vi "SVA 4MV6 T027 CCE.vi"(7 "NORMALIZACIÓN":bool, 8 "INVERTIDO?":bool, 9 "UMBRAL":u8(knob) scale=0.0..255.0, 10 "CAPA DE COLOR":T1(ring), 11 "RUTA DE IMAGEN":path) -> (2 "MOMENTOS INVARIANTES DE HU":dbl[](array[numeric]), 3 "IMAGEN BINARIZADA":picture)   [LabVIEW 2020]
doc: "Ceballos Conde Emanuel 4MV6 Sistemas de visión artificial 2022/1\nEste vi permite obtener una imagen binarizada y LOS SIETE MOMENTOS INVARIANTES DE HU de una imagen, tomando como referencia una de las capas seleccionadas."
panel:
  # "Ceballos Conde Emanuel\n4MV6\nSistemas de visión artificial\n2022/1"
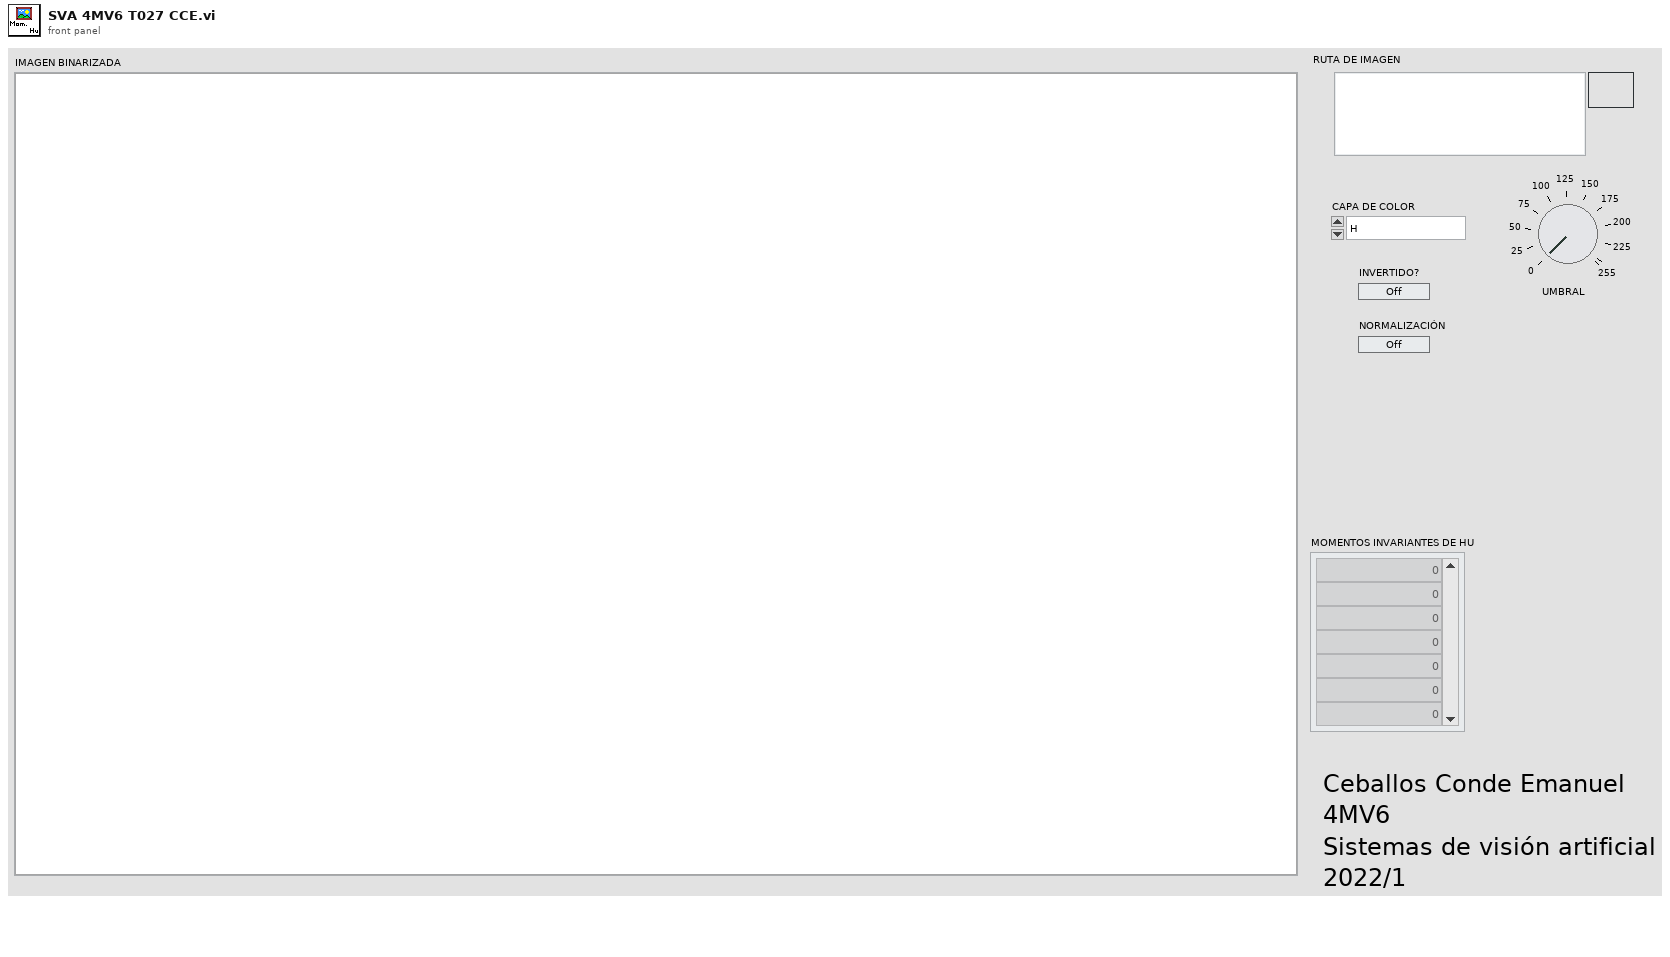
[diagram p1: front panel]
types:
  T1 = enum16{"H", "S", "V", "C", "M", "Y", "R", "G", "B", "RGB2GRAY MATLAB"}
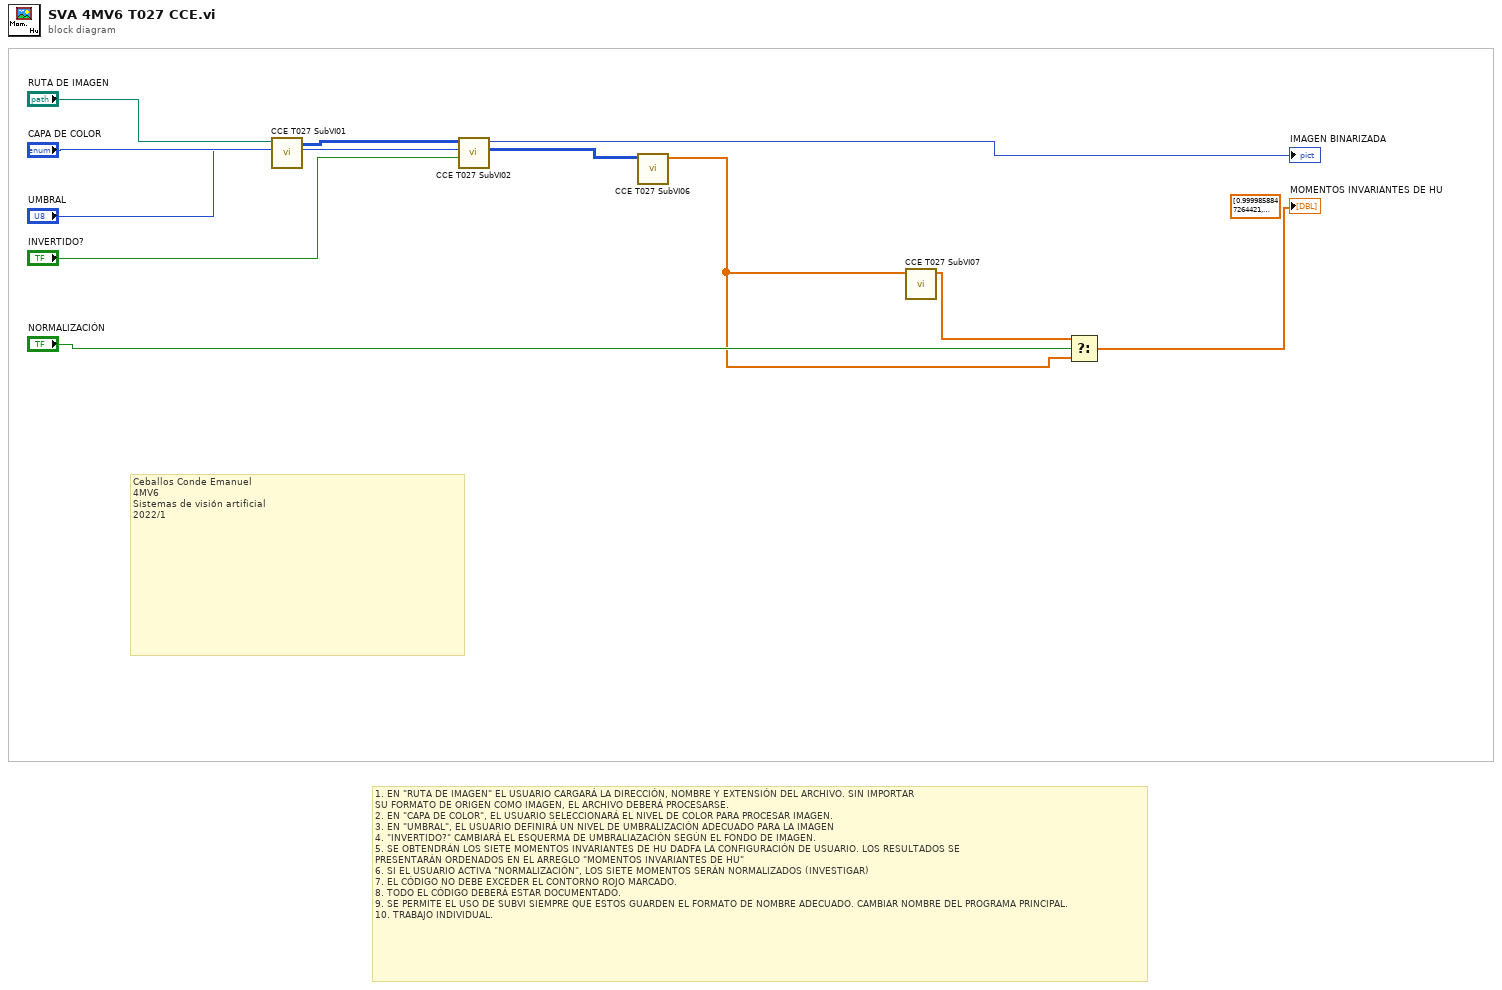
[diagram p0: block diagram]
diagram:
  (unwired) dbl[] [0.9999858847264421, 0.00020268683993240064, 0.0004447595314117563, 0.005290693434913511, -4.166575728385939e-06, -3.142609125743236e-07, -6.305309913794403e-07] ("MOMENTOS INVARIANTES DE HU")
  # "Ceballos Conde Emanuel\n4MV6\nSistemas de visión artificial\n2022/1"
  # "1. EN \"RUTA DE IMAGEN\" EL USUARIO CARGARÁ LA DIRECCIÓN, NOMBRE Y EXTENSIÓN DEL ARCHIVO. SIN IMPORTAR \nSU FORMATO DE ORIGEN COMO IMAGEN, EL ARCHIVO DEBERÁ PROCESARSE. \n2. EN \"CAPA DE COLOR\", EL USUARIO SELECCIONARÁ EL NIVEL DE COLOR PARA PROCESAR IMAGEN. \n3. EN \"UMBRAL\", EL USUARIO DEFINIRÁ UN NIVEL DE UMBRALIZACIÓN ADECUADO PARA LA IMAGEN \n4. \"INVERTIDO?\" CAMBIARÁ EL ESQUERMA DE UMBRALIAZACIÓN SEGÚN EL FONDO DE IMAGEN. \n5. SE OBTENDRÁN LOS SIETE MOMENTOS INVARIANTES DE HU DADFA LA CONFIGURACIÓN DE USUARIO. LOS RESULTADOS SE \nPRESENTARÁN ORDENADOS EN EL ARREGLO \"MOMENTOS INVARIANTES DE HU\"\n6. SI EL USUARIO ACTIVA \"NORMALIZACIÓN\", LOS SIETE MOMENTOS SERÁN NORMALIZADOS (INVESTIGAR) \n7. EL CÓDIGO NO DEBE EXCEDER EL CONTORNO ROJO MARCADO. \n8. TODO EL CÓDIGO DEBERÁ ESTAR DOCUMENTADO. \n9. SE PERMITE EL USO DE SUBVI SIEMPRE QUE ESTOS GUARDEN EL FORMATO DE NOMBRE ADECUADO. CAMBIAR NOMBRE DEL PROGRAMA PRINCIPAL. \n10. TRABAJO INDIVIDUAL."
  n1 = call "CCE T027 SubVI01.vi"("CAPA DE COLOR"="CAPA DE COLOR", "RUTA DE IMAGEN"="RUTA DE IMAGEN") -> ("Array"=w9:u8[][])  [unwired: 9 in]
  n2 = call "CCE T027 SubVI02.vi"("Array"=w9, "UMBRAL"="UMBRAL", "INVERTIDO?"="INVERTIDO?") -> ("new picture"=→"IMAGEN BINARIZADA":picture, "Array 2"=w5:u8[][])  [unwired: 6 in]
  n3 = call "CCE T027 SubVI06.vi"("Image Data"=w5) -> ("HU"=w2:dbl[])  [unwired: 10 in]
  n4 = call "CCE T027 SubVI07.vi"("array"=w2) -> ("normalizado"=w3:dbl[])  [unwired: 10 in]
  n5 = Select(t=w3, s="NORMALIZACIÓN", f=w2) -> (s? t:f=→"MOMENTOS INVARIANTES DE HU":dbl[])
